vi "Update Sensors.vi"(0 "RobotDriveDevRef":T1={"DevStatus"={"status"=FALSE, "code"=0, "source"=""}, "Motors[]"=[], "Square Inputs"=FALSE, "Max Output"=1.0}) -> (4 "Top Sensor":bool, 6 "Upper Sensor":bool, 8 "Middle Sensor":bool, 10 "Lower Sensor":bool, 15 "Bottom Sensor":bool)   [LabVIEW 2014]
uses:
  <vilib>/Rock Robotics/WPI/RobotDrive/WPI_RobotDriveDevRef.ctl
  <vilib>/Rock Robotics/WPI/MotorControl/WPI_MotorControlDeviceRef.ctl
  <vilib>/Rock Robotics/WPI/MotorControl/WPI_MotorControlType.ctl
  <vilib>/Rock Robotics/SystemInterfaces/Typedef/FPGA_TypedefDigitalModule.ctl
  <vilib>/Rock Robotics/SystemInterfaces/DIO/FPGA_DIOPWMChannel.ctl
  <vilib>/Rock Robotics/WPI/PWM/WPI_PWMDeadband.ctl
  <vilib>/Rock Robotics/WPI/CAN/Jaguar/SubVIs/WPI_CANJaguar_ControlMode.ctl
  <vilib>/Rock Robotics/WPI/CAN/TalonSRX/WPI_CANTalonSRX_APIControlMode.ctl
  <vilib>/Rock Robotics/WPI/PWM/WPI_PWMTransform_ConPane.ctl
  <vilib>/Rock Robotics/WPI/RobotDrive/WPI_RobotDriveMotorSelectorEnum.ctl
  Robot Global Data.vi
  <vilib>/Rock Robotics/Network Tables/SD Write Boolean.vi
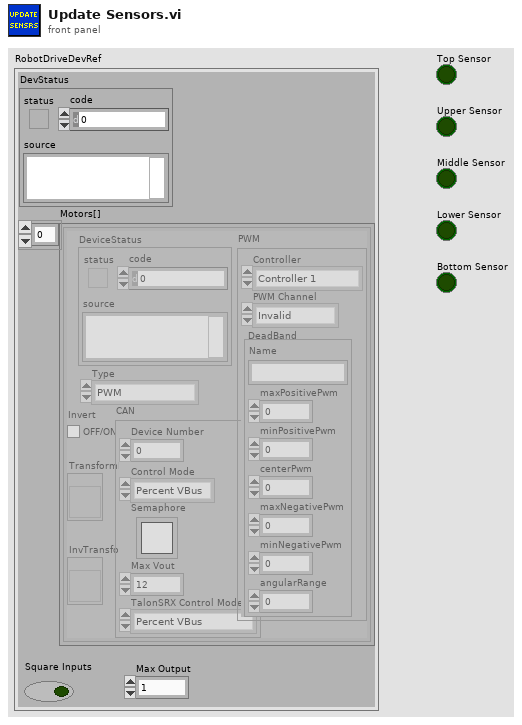
[diagram p1: front panel]
types:
  T1 = typedef "WPI_RobotDriveDevRef.ctl" = cluster{"DevStatus":errorcluster, "Motors[]":T2[], "Square Inputs":bool, "Max Output":dbl}
  T2 = typedef "WPI_MotorControlDeviceRef.ctl" = cluster{"DeviceStatus":errorcluster, "Type":T3, "PWM":cluster{"Controller":T4, "PWM Channel":T5, "DeadBand":T6}, "CAN":cluster{"Device Number":u8, "Control Mode":T7, "Semaphore":T8, "Max Vout":dbl, "TalonSRX Control Mode":T9}, "Invert":bool, "TransformRef":T10, "InvTransformRef":T10}
  T3 = typedef "WPI_MotorControlType.ctl" = enum16{"PWM", "CAN", "CANTalonSRX"}
  T4 = typedef "FPGA_TypedefDigitalModule.ctl" = enum16{"Controller 1"}
  T5 = typedef "FPGA_DIOPWMChannel.ctl" = enum8{"PWM 0", "PWM 1", "PWM 2", "PWM 3", "PWM 4", "PWM 5", "PWM 6", "PWM 7", "PWM 8", "PWM 9", "PWM MXP 0", "PWM MXP 1", "PWM MXP 2", "PWM MXP 3", "PWM MXP 4", "PWM MXP 5", "PWM MXP 6", "PWM MXP 7", "PWM MXP 8", "PWM MXP 9", "Invalid"}
  T6 = typedef "WPI_PWMDeadband.ctl" = cluster{"Name":string, "maxPositivePwm":i32, "minPositivePwm":i32, "centerPwm":i32, "maxNegativePwm":i32, "minNegativePwm":i32, "angularRange":u16}
  T7 = typedef "WPI_CANJaguar_ControlMode.ctl" = enum8{"Percent VBus", "Current", "Speed", "Position", "Voltage"}
  T8 = typedef "Semaphore RefNum" = refnum<k1>
  T9 = typedef "WPI_CANTalonSRX_APIControlMode.ctl" = enum8{"Percent VBus", "Speed", "Position", "Slave", "Unchanged / Invalid"}
  T10 = typedef "WPI_PWMTransform_ConPane.ctl" = refnum<vi>
  T11 = typedef "WPI_RobotDriveMotorSelectorEnum.ctl" = enum16{"Rear Left Motor", "Rear Right Motor", "Front Left Motor", "Front Right Motor"}
  T12 = typedef "WPI_SwitchDevRef.ctl" = cluster{"DevStatus":errorcluster, "DIO Channel":T13, "Controller":T4, "CntIndex":T14, "Normally Closed":bool}
  T13 = typedef "FPGA_DIOChannel.ctl" = enum8{"DIO 0", "DIO 1", "DIO 2", "DIO 3", "DIO 4", "DIO 5", "DIO 6", "DIO 7", "DIO 8", "DIO 9", "DIO MXP 0", "DIO MXP 1", "DIO MXP 2", "DIO MXP 3", "DIO MXP 4", "DIO MXP 5", "DIO MXP 6", "DIO MXP 7", "DIO MXP 8", "DIO MXP 9", "DIO MXP 10", "DIO MXP 11", "DIO MXP 12", "DIO MXP 13", "DIO MXP 14", "DIO MXP 15", "Invalid"}
  T14 = typedef "FPGA_CounterCtrSystemIndex.ctl" = enum8{"Ctr 0", "Ctr 1", "Ctr 2", "Ctr 3", "Ctr 4", "Ctr 5", "Ctr 6", "Ctr 7", "Invalid"}
  T15 = typedef "WPI_CANTalonSRX_GlobalStatus.ctl" = cluster{"Applied Throttle":dbl, "Module Enabled":bool, "CAN Error":errorcluster, "Closed Loop Error":dbl, "Forward Limit Switch Closed":bool, "Reverse Limit Switch Closed":bool, "Sensor Position":dbl, "Sensor Velocity":dbl, "Current":dbl, "Sticky Fault - Over Temp":bool, "Sticky Fault - Under Voltage":bool, "Sticky Fault - Forward Limit":bool, "Sticky Fault - Reverse Limit":bool, "Sticky Fault - Forward Soft Limit":bool, "Sticky Fault - Reverse Soft Limit":bool, "Brake is Enabled":bool, "Encoder Position":dbl, "Encoder Velocity":dbl, "Encoder Index Count":dbl, "Encoder A Pin State":bool, "Encoder B Pin State":bool, "Encoder Index Pin State":bool, "Analog In":dbl, "Analog In Velocity":dbl, "Temperature (C)":dbl, "Battery Voltage":dbl}
  T16 = cluster{"Encoders":cluster{"Drive Encoders":cluster{"Rear Left Motor":dbl, "Rear Right Motor":dbl, "Front Left Motor":dbl, "Front Right Motor":dbl}, "Other Encoders":cluster{"Lift":dbl}}}
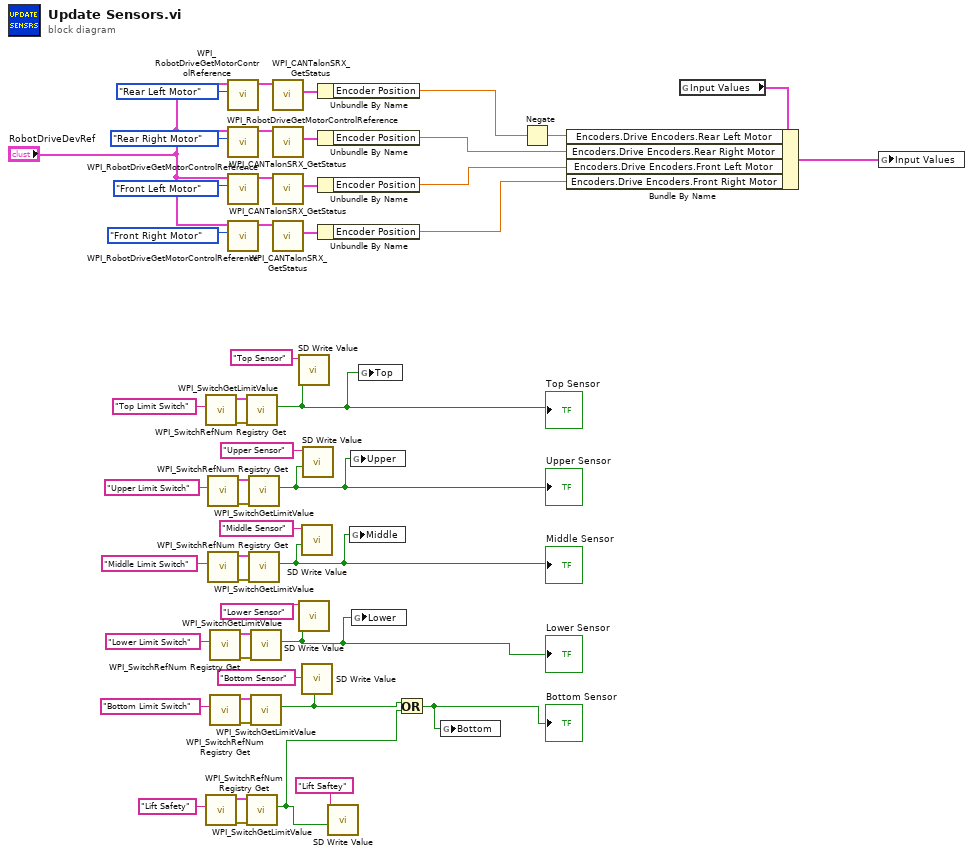
[diagram p0: block diagram]
diagram:
  n1 = call <vilib>:"WPI_SwitchRefNum Registry Get.vi"("refnum name"="Top Limit Switch") -> ("error out"=w15:errorcluster, "SwitchDevRef"=w14:T12)  [unwired: 9 in]
  n2 = call <vilib>:"WPI_SwitchRefNum Registry Get.vi"("refnum name"="Lift Safety") -> ("error out"=w9:errorcluster, "SwitchDevRef"=w8:T12)  [unwired: 9 in]
  n3 = call <vilib>:"WPI_SwitchRefNum Registry Get.vi"("refnum name"="Upper Limit Switch") -> ("error out"=w28:errorcluster, "SwitchDevRef"=w29:T12)  [unwired: 9 in]
  n4 = call <vilib>:"WPI_SwitchRefNum Registry Get.vi"("refnum name"="Middle Limit Switch") -> ("error out"=w25:errorcluster, "SwitchDevRef"=w26:T12)  [unwired: 9 in]
  n5 = call <vilib>:"WPI_SwitchRefNum Registry Get.vi"("refnum name"="Lower Limit Switch") -> ("error out"=w19:errorcluster, "SwitchDevRef"=w20:T12)  [unwired: 9 in]
  n6 = call <vilib>:"WPI_SwitchRefNum Registry Get.vi"("refnum name"="Bottom Limit Switch") -> ("error out"=w13:errorcluster, "SwitchDevRef"=w12:T12)  [unwired: 9 in]
  n7 = call <vilib>:"WPI_RobotDriveGetMotorControlReference.vi"("MotorIndex"=WPI_RobotDriveMotorSelectorEnum."Rear Left Motor", "RobotDriveDevRef"="RobotDriveDevRef") -> ("MotorControlDeviceRef"=w47:T2)  [unwired: 9 out]
  n8 = call <vilib>:"WPI_RobotDriveGetMotorControlReference.vi"("MotorIndex"=WPI_RobotDriveMotorSelectorEnum."Rear Right Motor", "RobotDriveDevRef"="RobotDriveDevRef") -> ("MotorControlDeviceRef"=w46:T2)  [unwired: 9 out]
  n9 = call <vilib>:"WPI_RobotDriveGetMotorControlReference.vi"("MotorIndex"=WPI_RobotDriveMotorSelectorEnum."Front Left Motor", "RobotDriveDevRef"="RobotDriveDevRef") -> ("MotorControlDeviceRef"=w45:T2)  [unwired: 9 out]
  n10 = call <vilib>:"WPI_RobotDriveGetMotorControlReference.vi"("MotorIndex"=WPI_RobotDriveMotorSelectorEnum."Front Right Motor", "RobotDriveDevRef"="RobotDriveDevRef") -> ("MotorControlDeviceRef"=w44:T2)  [unwired: 9 out]
  n11 = call <vilib>:"WPI_SwitchGetLimitValue.vi"("error in (no error)"=w15, "SwitchDevRef"=w14) -> ("Switch Pressed"=w5:bool)  [unwired: 7 in, 2 out]
  "Top Sensor" <- w5
  n12 = call <vilib>:"WPI_SwitchGetLimitValue.vi"("error in (no error)"=w9, "SwitchDevRef"=w8) -> ("Switch Pressed"=w31:bool)  [unwired: 7 in, 2 out]
  n13 = call <vilib>:"WPI_SwitchGetLimitValue.vi"("error in (no error)"=w28, "SwitchDevRef"=w29) -> ("Switch Pressed"=w4:bool)  [unwired: 7 in, 2 out]
  "Upper Sensor" <- w4
  n14 = call <vilib>:"WPI_SwitchGetLimitValue.vi"("error in (no error)"=w25, "SwitchDevRef"=w26) -> ("Switch Pressed"=w3:bool)  [unwired: 7 in, 2 out]
  "Middle Sensor" <- w3
  n15 = call <vilib>:"WPI_SwitchGetLimitValue.vi"("error in (no error)"=w19, "SwitchDevRef"=w20) -> ("Switch Pressed"=w2:bool)  [unwired: 7 in, 2 out]
  "Lower Sensor" <- w2
  n16 = call <vilib>:"WPI_SwitchGetLimitValue.vi"("error in (no error)"=w13, "SwitchDevRef"=w12) -> ("Switch Pressed"=w30:bool)  [unwired: 7 in, 2 out]
  n17 = call <vilib>:"WPI_CANTalonSRX_GetStatus.vi"("CAN Talon SRX Ref"=w47) -> ("Talon SRX Status"=w42:T15)  [unwired: 8 in, 2 out]
  n18 = call <vilib>:"WPI_CANTalonSRX_GetStatus.vi"("CAN Talon SRX Ref"=w46) -> ("Talon SRX Status"=w43:T15)  [unwired: 8 in, 2 out]
  n19 = call <vilib>:"WPI_CANTalonSRX_GetStatus.vi"("CAN Talon SRX Ref"=w45) -> ("Talon SRX Status"=w41:T15)  [unwired: 8 in, 2 out]
  n20 = call <vilib>:"WPI_CANTalonSRX_GetStatus.vi"("CAN Talon SRX Ref"=w44) -> ("Talon SRX Status"=w40:T15)  [unwired: 8 in, 2 out]
  n21 = call-poly <vilib>:"SD Write Value.vi"("Boolean"=w5, "Name"="Top Sensor") -> ()  [unwired: 8 in, 2 out]
  n22 = call-poly <vilib>:"SD Write Value.vi"("Boolean"=w2, "Name"="Lower Sensor") -> ()  [unwired: 8 in, 2 out]
  n23 = call-poly <vilib>:"SD Write Value.vi"("Boolean"=w3, "Name"="Middle Sensor") -> ()  [unwired: 8 in, 2 out]
  n24 = call-poly <vilib>:"SD Write Value.vi"("Boolean"=w30, "Name"="Bottom Sensor") -> ()  [unwired: 8 in, 2 out]
  n25 = call-poly <vilib>:"SD Write Value.vi"("Boolean"=w4, "Name"="Upper Sensor") -> ()  [unwired: 8 in, 2 out]
  n26 = Unbundle By Name(w42) -> ("Encoder Position"=w32:dbl)
  n27 = Unbundle By Name(w43) -> ("Encoder Position"=w39:dbl)
  n28 = Unbundle By Name(w41) -> ("Encoder Position"=w36:dbl)
  n29 = Unbundle By Name(w40) -> ("Encoder Position"=w34:dbl)
  n30 = call-poly <vilib>:"SD Write Value.vi"("Boolean"=w31, "Name"="Lift Saftey") -> ()  [unwired: 8 in, 2 out]
  n31 = global write "Robot Global Data.vi" "Middle"(w3) -> ()
  n32 = global write "Robot Global Data.vi" "Upper"(w4) -> ()
  n33 = global write "Robot Global Data.vi" "Lower"(w2) -> ()
  n34 = global write "Robot Global Data.vi" "Top"(w5) -> ()
  n35 = Or(x=w30, y=w31) -> (x .or. y?=w1:bool)
  "Bottom Sensor" <- w1
  n36 = global write "Robot Global Data.vi" "Bottom"(w1) -> ()
  n37 = Negate(x=w32) -> (-x=w33:dbl)
  n38 = global read "Robot Global Data.vi" "Input Values"() -> (w37:T16)
  n39 = Bundle By Name(cluster=w37, "Encoders.Drive Encoders.Rear Left Motor"=w33, "Encoders.Drive Encoders.Rear Right Motor"=w39, "Encoders.Drive Encoders.Front Left Motor"=w36, "Encoders.Drive Encoders.Front Right Motor"=w34) -> (w38:T16)
  n40 = global write "Robot Global Data.vi" "Input Values"(w38) -> ()
